vi "GenerareDateSimboluri.vi"() -> (0 "path":path)   [LabVIEW 2025]
uses:
  <vilib>/National Instruments/NI Super Simple Neural Networks/Types/Teaching Vector.ctl
  <vilib>/National Instruments/NI Super Simple Neural Networks/Types/1D Array.ctl
  <vilib>/National Instruments/NI Super Simple Neural Networks/Neural Network.lvclass
panel:
  out "error out":errorcluster
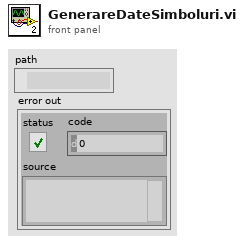
[diagram p1: front panel]
types:
  T1 = typedef "Neural Network.lvclass/Teaching Vector.ctl" = cluster{"Inputs":T2, "Expected Outputs":T2}
  T2 = typedef "Neural Network.lvclass/1D Array.ctl" = cluster{"1D Array":dbl[]}
  T3 = enum16{"open", "replace", "create", "open or create", "replace or create", "replace or create with confirmation"}
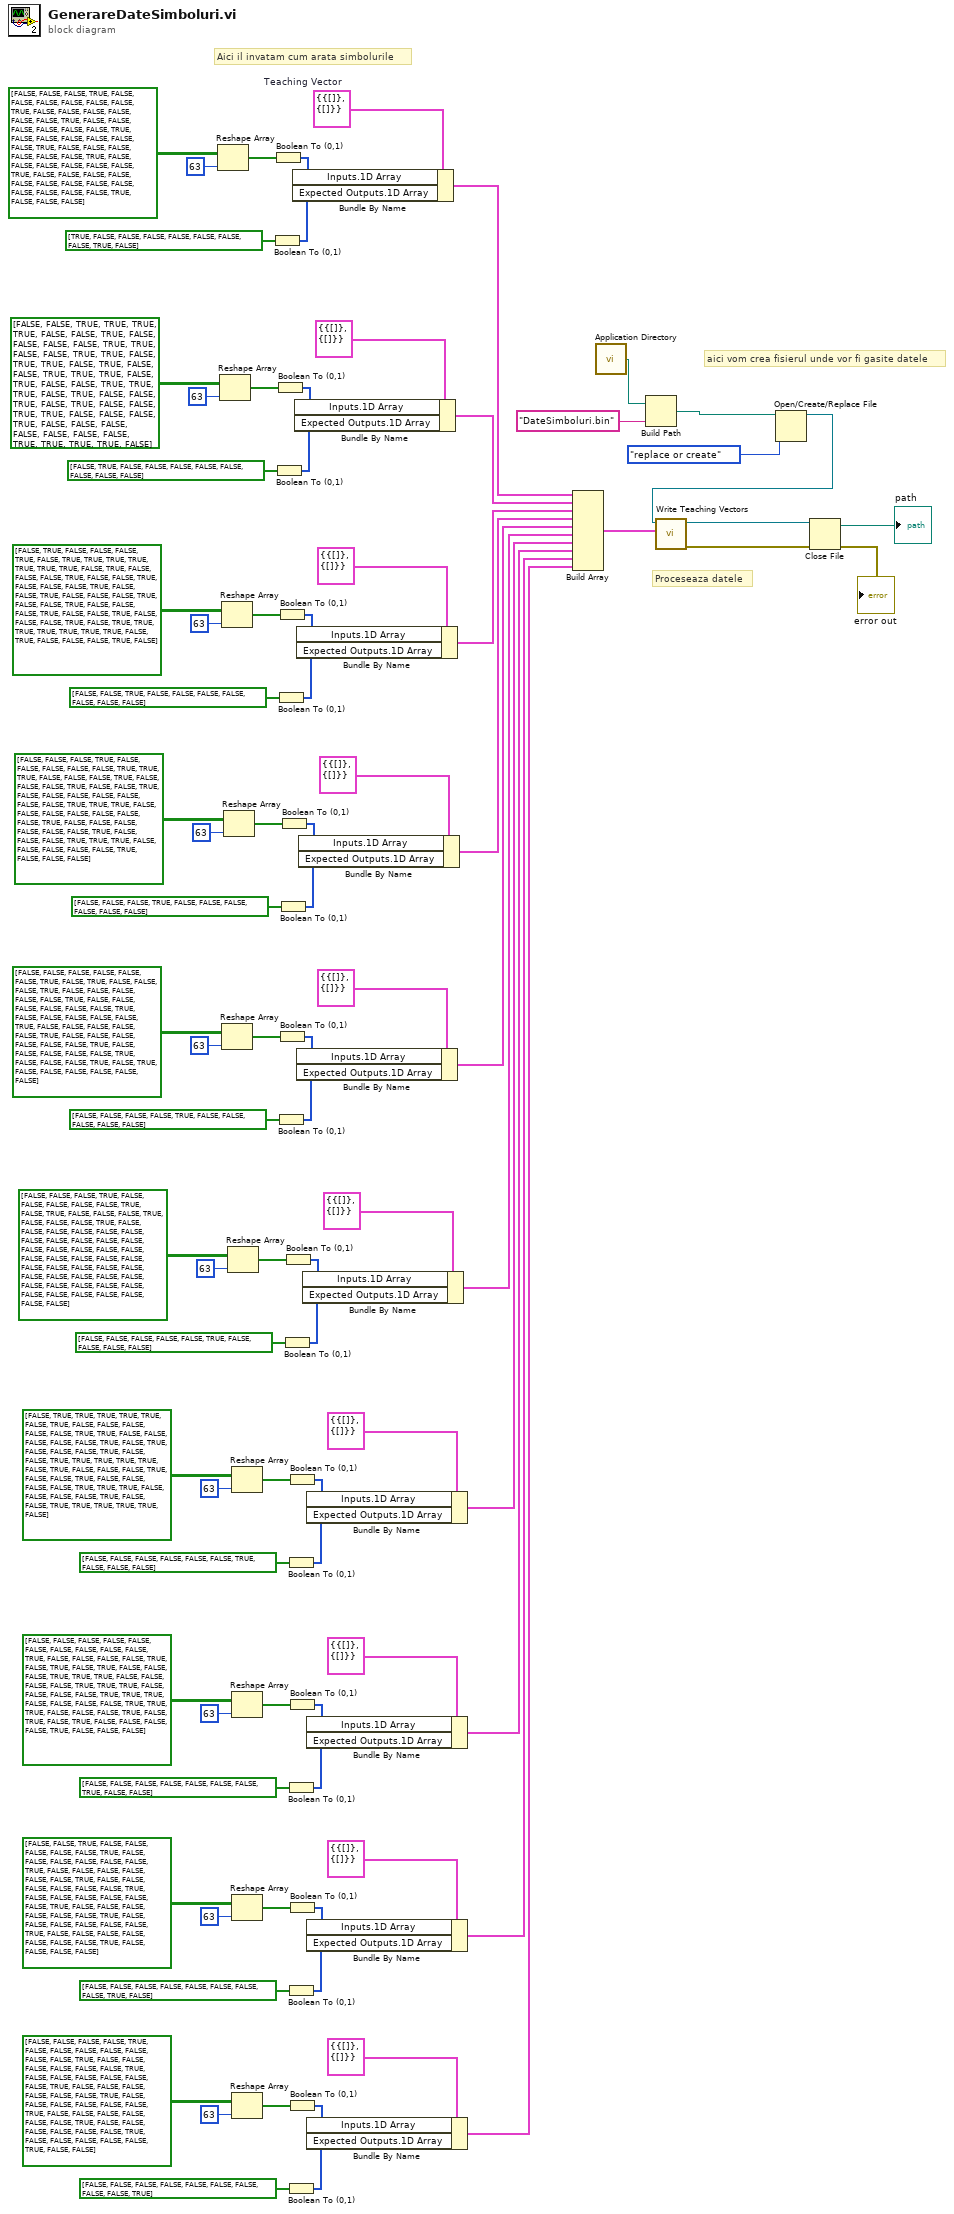
[diagram p0: block diagram]
diagram:
  w86 = T1 {"Inputs"={"1D Array"=[]}, "Expected Outputs"={"1D Array"=[]}}  # Teaching Vector
  # "Proceseaza datele"
  # "aici vom crea fisierul unde vor fi gasite datele"
  # "Aici il invatam cum arata simbolurile"
  n1 = Reshape Array(bool[][] [[FALSE, FALSE, FALSE, TRUE, FALSE, FALSE, FALSE], [FALSE, FALSE, FALSE, TRUE, FALSE, FALSE, FALSE], [FALSE, FALSE, FALSE, TRUE, FALSE, FALSE, FALSE], [FALSE, FALSE, FALSE, TRUE, FALSE, FALSE, FALSE], [FALSE, FALSE, FALSE, TRUE, FALSE, FALSE, FALSE], [FALSE, FALSE, FALSE, TRUE, FALSE, FALSE, FALSE], [FALSE, FALSE, FALSE, TRUE, FALSE, FALSE, FALSE], [FALSE, FALSE, FALSE, FALSE, FALSE, FALSE, FALSE], [FALSE, FALSE, FALSE, TRUE, FALSE, FALSE, FALSE]], 63 ("dimension size")) -> (w88:bool[])
  n2 = Reshape Array(bool[][] [[FALSE, FALSE, TRUE, TRUE, TRUE, TRUE, FALSE], [FALSE, TRUE, FALSE, FALSE, FALSE, FALSE, TRUE], [TRUE, FALSE, FALSE, TRUE, TRUE, FALSE, TRUE], [TRUE, FALSE, TRUE, FALSE, FALSE, TRUE, TRUE], [TRUE, FALSE, TRUE, FALSE, FALSE, TRUE, TRUE], [TRUE, FALSE, TRUE, FALSE, FALSE, TRUE, FALSE], [TRUE, FALSE, FALSE, TRUE, TRUE, FALSE, FALSE], [FALSE, TRUE, FALSE, FALSE, FALSE, FALSE, FALSE], [FALSE, FALSE, TRUE, TRUE, TRUE, TRUE, FALSE]], 63 ("dimension size")) -> (w72:bool[])
  n3 = Reshape Array(bool[][] [[FALSE, TRUE, FALSE, FALSE, FALSE, TRUE, FALSE], [TRUE, TRUE, TRUE, TRUE, TRUE, TRUE, TRUE], [FALSE, TRUE, FALSE, FALSE, FALSE, TRUE, FALSE], [FALSE, TRUE, FALSE, FALSE, FALSE, TRUE, FALSE], [FALSE, TRUE, FALSE, FALSE, FALSE, TRUE, FALSE], [FALSE, TRUE, FALSE, FALSE, FALSE, TRUE, FALSE], [FALSE, TRUE, FALSE, FALSE, FALSE, TRUE, FALSE], [TRUE, TRUE, TRUE, TRUE, TRUE, TRUE, TRUE], [FALSE, TRUE, FALSE, FALSE, FALSE, TRUE, FALSE]], 63 ("dimension size")) -> (w65:bool[])
  n4 = Reshape Array(bool[][] [[FALSE, FALSE, FALSE, FALSE, FALSE, FALSE, TRUE], [FALSE, TRUE, FALSE, FALSE, FALSE, TRUE, FALSE], [FALSE, FALSE, FALSE, FALSE, TRUE, FALSE, FALSE], [FALSE, FALSE, FALSE, FALSE, TRUE, FALSE, FALSE], [FALSE, FALSE, FALSE, TRUE, FALSE, FALSE, FALSE], [FALSE, FALSE, TRUE, FALSE, FALSE, FALSE, FALSE], [FALSE, FALSE, TRUE, FALSE, FALSE, FALSE, FALSE], [FALSE, TRUE, FALSE, FALSE, FALSE, TRUE, FALSE], [TRUE, FALSE, FALSE, FALSE, FALSE, FALSE, FALSE]], 63 ("dimension size")) -> (w51:bool[])
  n5 = Reshape Array(bool[][] [[FALSE, FALSE, FALSE, TRUE, FALSE, FALSE, FALSE], [FALSE, FALSE, TRUE, TRUE, TRUE, FALSE, FALSE], [FALSE, TRUE, FALSE, FALSE, FALSE, TRUE, FALSE], [FALSE, TRUE, FALSE, FALSE, FALSE, FALSE, FALSE], [FALSE, FALSE, TRUE, TRUE, TRUE, FALSE, FALSE], [FALSE, FALSE, FALSE, FALSE, FALSE, TRUE, FALSE], [FALSE, FALSE, FALSE, FALSE, FALSE, TRUE, FALSE], [FALSE, FALSE, TRUE, TRUE, TRUE, FALSE, FALSE], [FALSE, FALSE, FALSE, TRUE, FALSE, FALSE, FALSE]], 63 ("dimension size")) -> (w58:bool[])
  n6 = Reshape Array(bool[][] [[FALSE, FALSE, FALSE, TRUE, FALSE, FALSE, FALSE], [FALSE, FALSE, TRUE, FALSE, TRUE, FALSE, FALSE], [FALSE, TRUE, FALSE, FALSE, FALSE, TRUE, FALSE], [FALSE, FALSE, FALSE, FALSE, FALSE, FALSE, FALSE], [FALSE, FALSE, FALSE, FALSE, FALSE, FALSE, FALSE], [FALSE, FALSE, FALSE, FALSE, FALSE, FALSE, FALSE], [FALSE, FALSE, FALSE, FALSE, FALSE, FALSE, FALSE], [FALSE, FALSE, FALSE, FALSE, FALSE, FALSE, FALSE], [FALSE, FALSE, FALSE, FALSE, FALSE, FALSE, FALSE]], 63 ("dimension size")) -> (w44:bool[])
  n7 = Reshape Array(bool[][] [[FALSE, TRUE, TRUE, TRUE, TRUE, TRUE, FALSE], [TRUE, FALSE, FALSE, FALSE, FALSE, FALSE, TRUE], [TRUE, FALSE, FALSE, FALSE, FALSE, FALSE, TRUE], [FALSE, TRUE, FALSE, FALSE, FALSE, TRUE, FALSE], [FALSE, TRUE, TRUE, TRUE, TRUE, TRUE, FALSE], [TRUE, FALSE, FALSE, FALSE, TRUE, FALSE, FALSE], [TRUE, FALSE, FALSE, FALSE, FALSE, TRUE, TRUE], [TRUE, FALSE, FALSE, FALSE, FALSE, TRUE, FALSE], [FALSE, TRUE, TRUE, TRUE, TRUE, TRUE, FALSE]], 63 ("dimension size")) -> (w37:bool[])
  n8 = Reshape Array(bool[][] [[FALSE, FALSE, FALSE, FALSE, FALSE, FALSE, FALSE], [FALSE, FALSE, FALSE, TRUE, FALSE, FALSE, FALSE], [FALSE, TRUE, FALSE, TRUE, FALSE, TRUE, FALSE], [FALSE, FALSE, TRUE, TRUE, TRUE, FALSE, FALSE], [FALSE, FALSE, TRUE, TRUE, TRUE, FALSE, FALSE], [FALSE, FALSE, TRUE, TRUE, TRUE, FALSE, FALSE], [FALSE, FALSE, TRUE, TRUE, TRUE, FALSE, FALSE], [FALSE, TRUE, FALSE, TRUE, FALSE, TRUE, FALSE], [FALSE, FALSE, FALSE, TRUE, FALSE, FALSE, FALSE]], 63 ("dimension size")) -> (w30:bool[])
  n9 = Reshape Array(bool[][] [[FALSE, FALSE, TRUE, FALSE, FALSE, FALSE, FALSE], [FALSE, TRUE, FALSE, FALSE, FALSE, FALSE, FALSE], [FALSE, TRUE, FALSE, FALSE, FALSE, FALSE, FALSE], [FALSE, TRUE, FALSE, FALSE, FALSE, FALSE, FALSE], [FALSE, TRUE, FALSE, FALSE, FALSE, FALSE, FALSE], [FALSE, TRUE, FALSE, FALSE, FALSE, FALSE, FALSE], [FALSE, TRUE, FALSE, FALSE, FALSE, FALSE, FALSE], [FALSE, TRUE, FALSE, FALSE, FALSE, FALSE, FALSE], [FALSE, FALSE, TRUE, FALSE, FALSE, FALSE, FALSE]], 63 ("dimension size")) -> (w23:bool[])
  n10 = Reshape Array(bool[][] [[FALSE, FALSE, FALSE, FALSE, TRUE, FALSE, FALSE], [FALSE, FALSE, FALSE, FALSE, FALSE, TRUE, FALSE], [FALSE, FALSE, FALSE, FALSE, FALSE, TRUE, FALSE], [FALSE, FALSE, FALSE, FALSE, FALSE, TRUE, FALSE], [FALSE, FALSE, FALSE, FALSE, FALSE, TRUE, FALSE], [FALSE, FALSE, FALSE, FALSE, FALSE, TRUE, FALSE], [FALSE, FALSE, FALSE, FALSE, FALSE, TRUE, FALSE], [FALSE, FALSE, FALSE, FALSE, FALSE, TRUE, FALSE], [FALSE, FALSE, FALSE, FALSE, TRUE, FALSE, FALSE]], 63 ("dimension size")) -> (w16:bool[])
  n11 = Boolean To (0,1)(Boolean=bool[] [TRUE, FALSE, FALSE, FALSE, FALSE, FALSE, FALSE, FALSE, TRUE, FALSE]) -> (0, 1=w84:i16[])
  n12 = Boolean To (0,1)(Boolean=w88) -> (0, 1=w85:i16[])
  n13 = Boolean To (0,1)(Boolean=bool[] [FALSE, TRUE, FALSE, FALSE, FALSE, FALSE, FALSE, FALSE, FALSE, FALSE]) -> (0, 1=w68:i16[])
  n14 = Boolean To (0,1)(Boolean=w72) -> (0, 1=w69:i16[])
  n15 = Boolean To (0,1)(Boolean=bool[] [FALSE, FALSE, TRUE, FALSE, FALSE, FALSE, FALSE, FALSE, FALSE, FALSE]) -> (0, 1=w61:i16[])
  n16 = Boolean To (0,1)(Boolean=bool[] [FALSE, FALSE, FALSE, FALSE, TRUE, FALSE, FALSE, FALSE, FALSE, FALSE]) -> (0, 1=w47:i16[])
  n17 = Boolean To (0,1)(Boolean=w65) -> (0, 1=w62:i16[])
  n18 = Boolean To (0,1)(Boolean=w51) -> (0, 1=w48:i16[])
  n19 = Boolean To (0,1)(Boolean=bool[] [FALSE, FALSE, FALSE, TRUE, FALSE, FALSE, FALSE, FALSE, FALSE, FALSE]) -> (0, 1=w54:i16[])
  n20 = Boolean To (0,1)(Boolean=w58) -> (0, 1=w55:i16[])
  n21 = Boolean To (0,1)(Boolean=bool[] [FALSE, FALSE, FALSE, FALSE, FALSE, TRUE, FALSE, FALSE, FALSE, FALSE]) -> (0, 1=w40:i16[])
  n22 = Boolean To (0,1)(Boolean=w44) -> (0, 1=w41:i16[])
  n23 = Boolean To (0,1)(Boolean=bool[] [FALSE, FALSE, FALSE, FALSE, FALSE, FALSE, TRUE, FALSE, FALSE, FALSE]) -> (0, 1=w33:i16[])
  n24 = Boolean To (0,1)(Boolean=bool[] [FALSE, FALSE, FALSE, FALSE, FALSE, FALSE, FALSE, TRUE, FALSE, FALSE]) -> (0, 1=w26:i16[])
  n25 = Boolean To (0,1)(Boolean=bool[] [FALSE, FALSE, FALSE, FALSE, FALSE, FALSE, FALSE, FALSE, TRUE, FALSE]) -> (0, 1=w19:i16[])
  n26 = Boolean To (0,1)(Boolean=bool[] [FALSE, FALSE, FALSE, FALSE, FALSE, FALSE, FALSE, FALSE, FALSE, TRUE]) -> (0, 1=w12:i16[])
  n27 = Boolean To (0,1)(Boolean=w37) -> (0, 1=w34:i16[])
  n28 = Boolean To (0,1)(Boolean=w30) -> (0, 1=w27:i16[])
  n29 = Boolean To (0,1)(Boolean=w23) -> (0, 1=w20:i16[])
  n30 = Boolean To (0,1)(Boolean=w16) -> (0, 1=w13:i16[])
  n31 = Bundle By Name "Bundle By Name"(cluster=w86, "Inputs.1D Array"=w85, "Expected Outputs.1D Array"=w84) -> (w83:T1)
  n32 = Bundle By Name(cluster=T1 {"Inputs"={"1D Array"=[]}, "Expected Outputs"={"1D Array"=[]}} ("Teaching Vector"), "Inputs.1D Array"=w69, "Expected Outputs.1D Array"=w68) -> (w11:T1)
  n33 = Bundle By Name(cluster=T1 {"Inputs"={"1D Array"=[]}, "Expected Outputs"={"1D Array"=[]}} ("Teaching Vector"), "Inputs.1D Array"=w62, "Expected Outputs.1D Array"=w61) -> (w10:T1)
  n34 = Bundle By Name(cluster=T1 {"Inputs"={"1D Array"=[]}, "Expected Outputs"={"1D Array"=[]}} ("Teaching Vector"), "Inputs.1D Array"=w48, "Expected Outputs.1D Array"=w47) -> (w8:T1)
  n35 = Bundle By Name(cluster=T1 {"Inputs"={"1D Array"=[]}, "Expected Outputs"={"1D Array"=[]}} ("Teaching Vector"), "Inputs.1D Array"=w55, "Expected Outputs.1D Array"=w54) -> (w9:T1)
  n36 = Bundle By Name(cluster=T1 {"Inputs"={"1D Array"=[]}, "Expected Outputs"={"1D Array"=[]}} ("Teaching Vector"), "Inputs.1D Array"=w41, "Expected Outputs.1D Array"=w40) -> (w7:T1)
  n37 = Bundle By Name(cluster=T1 {"Inputs"={"1D Array"=[]}, "Expected Outputs"={"1D Array"=[]}} ("Teaching Vector"), "Inputs.1D Array"=w34, "Expected Outputs.1D Array"=w33) -> (w6:T1)
  n38 = Bundle By Name(cluster=T1 {"Inputs"={"1D Array"=[]}, "Expected Outputs"={"1D Array"=[]}} ("Teaching Vector"), "Inputs.1D Array"=w27, "Expected Outputs.1D Array"=w26) -> (w5:T1)
  n39 = Bundle By Name(cluster=T1 {"Inputs"={"1D Array"=[]}, "Expected Outputs"={"1D Array"=[]}} ("Teaching Vector"), "Inputs.1D Array"=w20, "Expected Outputs.1D Array"=w19) -> (w4:T1)
  n40 = Bundle By Name(cluster=T1 {"Inputs"={"1D Array"=[]}, "Expected Outputs"={"1D Array"=[]}} ("Teaching Vector"), "Inputs.1D Array"=w13, "Expected Outputs.1D Array"=w12) -> (w3:T1)
  n41 = Build Array "Build Array"(w83, w11, w10, w9, w8, w7, w6, w5, w4, w3) -> (w82:T1[])
  n42 = call <vilib>:"Application Directory.vi"() -> ("Application Directory"=w81:path)
  n43 = Build Path(base path=w81, name or relative path="DateSimboluri.bin") -> (appended path=w1:path)
  n44 = Open/Create/Replace File(file path (use dialog)=w1, operation (0:open)=T3."replace or create") -> (refnum out=w2:refnum<file>)  [unwired: 4 in, 2 out]
  n45 = call <vilib>:"Write Teaching Vectors.vi"("Teaching Vectors"=w82, "Teaching File Ref In"=w2) -> ("Error Out"=w77:errorcluster, "Teaching File Ref Out"=w78:refnum<file>)  [unwired: 8 in]
  n46 = Close File(refnum=w78, error in=w77) -> (path=→"path":path, error out=→"error out":errorcluster)
